vi "Test Minimal Audio Device Playback.vi"(8 "error in (no error)":errorcluster) -> (0 "error out":errorcluster, 3 "Pass?":bool)   [LabVIEW 2020]
uses:
  G-Audio/Audio Files/Polymorphic VIs/Quick Load Audio File (Path).vi
  678bb3a3-ab52-4f1b-8279-67e7041d0764.vi
  G-Audio/Private/Path To UTF-8 String.vi
  G-Audio/Audio Files/Private/Quick Load Audio File (Core).vi
  G-Audio/Private/Result To Error.vi
  678bb3a3-ab52-4f1b-8279-67e7041d0764.vi/4dfb5711-8d81-45a3-b3db-a84d40650863.vi
  678bb3a3-ab52-4f1b-8279-67e7041d0764.vi/c8869513-30c6-44f2-a2d3-73232fe63870.vi
  678bb3a3-ab52-4f1b-8279-67e7041d0764.vi/4dfb5711-8d81-45a3-b3db-a84d40650863.vi/4b7b629c-2e91-4160-9820-a26af8f6e677.vi
  678bb3a3-ab52-4f1b-8279-67e7041d0764.vi/c8869513-30c6-44f2-a2d3-73232fe63870.vi/4b7b629c-2e91-4160-9820-a26af8f6e677.vi
  <vilib>/Utility/error.llb/Error Cluster From Error Code.vi
  G-Audio/Private/Copy Data.vi
  <vilib>/Utility/Data Type/Get Numeric Information.vi
  G-Audio/G-Audio.lvlib
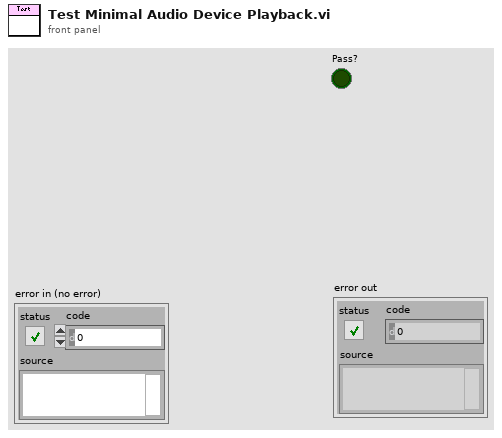
[diagram p1: front panel]
types:
  T1 = typedef "G-Audio.lvlib/Audio Device Refnum.ctl" = refnum<file>
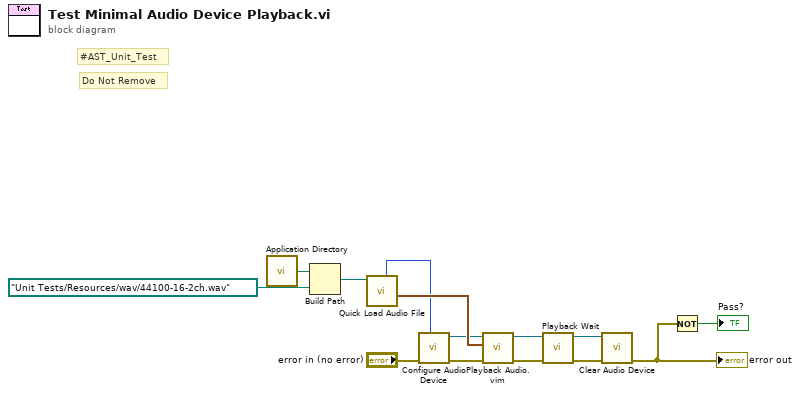
[diagram p0: block diagram]
diagram:
  # "Do Not Remove"
  # "#AST_Unit_Test"
  n1 = call <vilib>:"Application Directory.vi"() -> ("Application Directory"=w14:path)
  n2 = Build Path(base path=w14, name or relative path=path "Unit Tests/Resources/wav/44100-16-2ch.wav" ("Path")) -> (appended path=w12:path)
  n3 = call-poly "Quick Load Audio File.vi"("Path"=w12) -> ("data"=w11:waveform(i16)[], "PCM Frame Length"=w10:u64)  [unwired: 5 in, 4 out]
  n4 = call "Configure Audio Device.vi"("Buffer Size (4096)"=w10, "error in (no error)"="error in (no error)") -> ("error out"=w7:errorcluster, "Audio Device Refnum"=w8:T1)  [unwired: 8 in]
  n5 = call "Playback Audio.vim"("error in (no error)"=w7, "Audio Data"=w11, "Audio Device Refnum In"=w8) -> ("error out"=w4:errorcluster, "Audio Device Refnum Out"=w6:T1)  [unwired: 7 in]
  n6 = call "Playback Wait.vi"("error in (no error)"=w4, "Audio Device Refnum In"=w6) -> ("error out"=w3:errorcluster, "Audio Device Refnum Out"=w5:T1)  [unwired: 8 in]
  n7 = call "Clear Audio Device.vi"("error in (no error)"=w3, "Audio Device Refnum In"=w5) -> ("error out"=w1:errorcluster)  [unwired: 9 in]
  "error out" <- w1
  n8 = Not(x=w1) -> (.not. x?=→"Pass?":bool)
